vi "UnitatsStringsValors.vi"(2 "UnitatsC1":string, 3 "Arr Refnum":refnum<vi>) -> (0 "Array":cluster{"String":string, "Value":u16}[](array[cluster]), 1 "Array 2":cluster{"String":string, "Value":u16}[](array[cluster]))   [LabVIEW 2017]
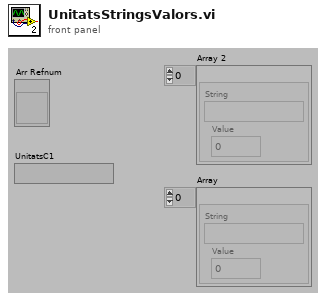
[diagram p1: front panel]
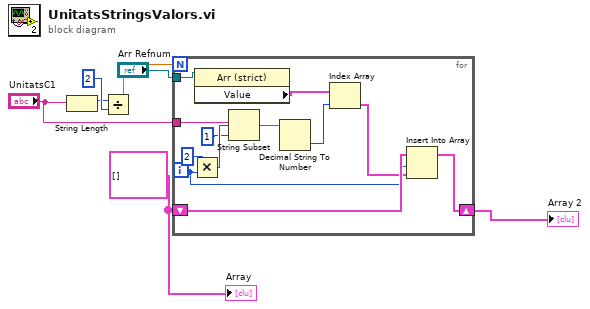
[diagram p0: block diagram]
diagram:
  w6 = cluster{"String":string, "Value":u16}[] []
  n1 = String Length(string="UnitatsC1") -> (length=w2:i32)
  n2 = Divide(x=w2, y=2) -> (x/y=w4:dbl)
  n3 = for {
    N: w4 -> [_]
    tunnel: "UnitatsC1" -> [w19]
    shift-right: [w14] -> w5
    shift-left: w6 -> [w13]
    tunnel: "Arr Refnum" -> [w8]
    i -> [w12]
    n4 = Multiply(x=u8 2, y=w12) -> (x*y=w16:i32)
    n5 = property on="Property Node" class="Arr (strict)"(reference=w8) -> ("Value"=w11:cluster{"String":string, "Value":u16}[])  [unwired: 1 in, 2 out]
    n6 = String Subset(string=w19, offset (0)=w16, length (rest)=1 ("length (rest)")) -> (substring=w18:string)
    n7 = Decimal String To Number(string=w18) -> (number=w10:i32)  [unwired: 2 in, 1 out]
    n8 = Index Array(array=w11, index=w10) -> (element=w9:cluster{"String":string, "Value":u16})
    n9 = Insert Into Array(array=w13, index=w12, new element=w9) -> (w14:cluster{"String":string, "Value":u16}[])
  }
  "Array 2" <- w5
  "Array" <- w6
